vi "Stop Panel.vi"(6 "Panel Host":refnum<vi>, 8 "error in (no error)":errorcluster, 9 "Panel":enum16{"Input Panel", "Output Panel"}(ring), 10 "Panel VI in":refnum<vi>, 11 "CallVIStep in":refnum<class "CallVIStep.lvclass">) -> (0 "error out":errorcluster, 3 "CallVIStep out":refnum<class "CallVIStep.lvclass">)   [LabVIEW 2015, in "CallVIStep.lvclass"]
uses:
  CallVIStep.lvclass
  Step.lvclass
  Project.lvclass
  Editor/Editor.lvclass
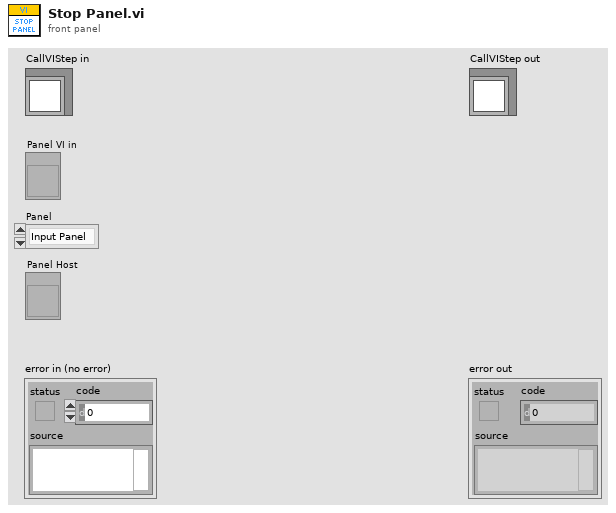
[diagram p1: front panel]
types:
  T1 = typedef "Step.lvclass/STEP_OUTPUT.ctl" = cluster{"Label":string, "Name":string, "Data Type":T2, "Check Type":T3, "String Limit":string, "Lower Limit":dbl, "Upper Limit":dbl, "Boolean Limit":bool, "Ignore Case":bool, "Variable Name 1":string, "Limit Value Type 1":T4, "Variable Name 2":string, "Limit Value Type 2":T4}
  T2 = typedef "Step.lvclass/OUTPUT_DATA_TYPE.ctl" = enum16{"Boolean", "String", "Numeric", "Other"}
  T3 = typedef "Step.lvclass/OUTPUT_CHECK_TYPE.ctl" = enum16{"INVALID", "DO_NOT_CHECK", "RECORD", "VARIABLE", "EQUAL", "NOT_EQUAL", "STR_CONTAINS", "STR_START_WITH", "STR_END_WITH", "STR_REGEX_MATCH", "NUM_GT", "NUM_LT", "NUM_GE", "NUM_LE", "NUM_RANGE", "NUM_RANGE_BDY"}
  T4 = typedef "Step.lvclass/OUTPUT_VALUE_TYPE.ctl" = enum16{"Constant", "Variable"}
  T5 = typedef "CallVIStep.lvclass/VI Input Typedef.ctl" = cluster{"Label":string, "Input Type":T6, "Type String":i16[], "Data String":string, "Variable Name":string}
  T6 = typedef "CallVIStep.lvclass/VI Input Type Typedef.ctl" = enum16{"Default", "Value", "Variable"}
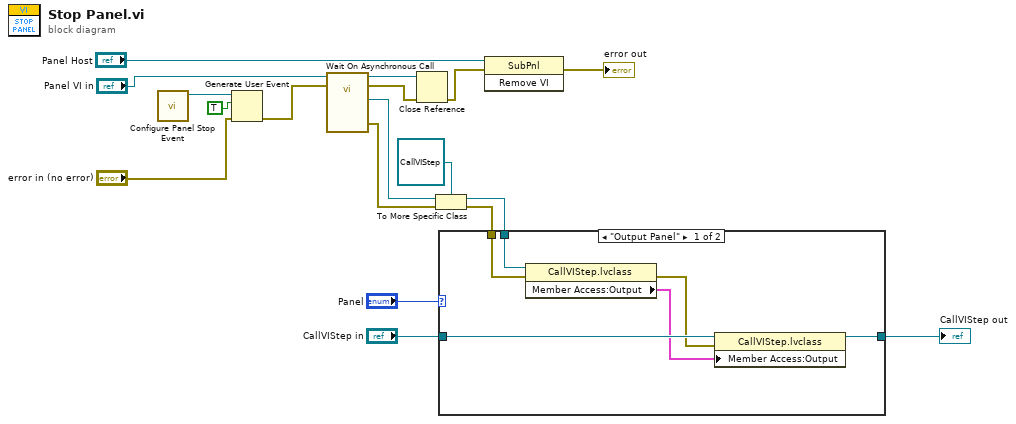
[diagram p0: block diagram]
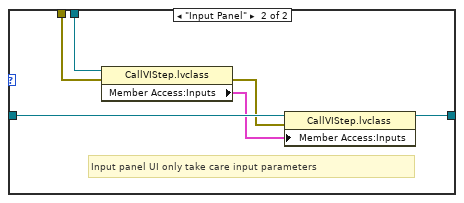
[diagram p2: hidden frame]
diagram:
  n1 = call "Configure Panel Stop Event.vi"() -> ("Panel Stop event"=w14:refnum<user-event>)  [unwired: 11 in]
  n2 = Generate User Event(user event=w14, event data cluster=TRUE, error in="error in (no error)") -> (error out=w12:errorcluster)  [unwired: 1 in, 1 out]
  n3 = call-by-ref "Wait On Asynchronous Call"(reference="Panel VI in", error in=w12) -> (reference out=w18:refnum<vi>, error out=w17:errorcluster, 0:"error out"=w5:errorcluster, "Step out"=w4:refnum<class "Step.lvclass">)  [unwired: 10 in]
  n4 = Close Reference(reference=w18, error in (no error)=w17) -> (error out=w11:errorcluster)
  n5 = To More Specific Class(target class=refnum<class "CallVIStep.lvclass"> refnum ("CallVIStep in"), reference=w4, error in=w5) -> (specific class reference=w1:refnum<class "CallVIStep.lvclass">, error out=w2:errorcluster)
  n6 = case shown="\"Output Panel\"" "Panel" {
    tunnel: w1 -> [w24 w30]
    tunnel: w2 -> [w23 w29]
    tunnel: "CallVIStep in" -> [w22 w28]
    tunnel: [w20 w26] -> w7
    frame "Output Panel" {
      n7 = property class="CallVIStep.lvclass"(reference=w24, error in=w23) -> (error out=w19:errorcluster, "Member Access:Output"=w21:T1[])  [unwired: 1 out]
      n8 = property class="CallVIStep.lvclass"(reference=w22, error in=w19, "Member Access:Output"=w21) -> (reference out=w20:refnum<class "CallVIStep.lvclass">)  [unwired: 1 out]
    }
    frame "Input Panel" {
      # "Input panel UI only take care input parameters"
      n9 = property class="CallVIStep.lvclass"(reference=w30, error in=w29) -> (error out=w25:errorcluster, "Member Access:Inputs"=w27:T5[])  [unwired: 1 out]
      n10 = property class="CallVIStep.lvclass"(reference=w28, error in=w25, "Member Access:Inputs"=w27) -> (reference out=w26:refnum<class "CallVIStep.lvclass">)  [unwired: 1 out]
    }
  }
  "CallVIStep out" <- w7
  n11 = invoke class="SubPnl" method="Remove VI"(reference="Panel Host", error in=w11) -> (error out=→"error out":errorcluster)  [unwired: 1 in, 2 out]
